vi "CRYMake CRY6181 Calibration Data.vi"() -> (0 "Error":bool)   [LabVIEW 2013]
uses:
  Typedef Control/CRYHardware Channel Info.ctl
  Typedef Control/CRYCalibration 2DCluster.ctl
  Typedef Control/CRYCalibration Cluster.ctl
  Typedef Control/CRYData Cluster.ctl
  CRYProject/CRYProject Editor Global.vi
  Calibration/SubVI/CRYCal Global.vi
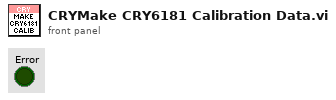
[diagram p1: front panel]
types:
  T1 = typedef "CRYCalibration 2DCluster.ctl" = cluster{"Calibration":T2, "Corr Curve":T3, "EQ Curve":T3, "Sens Curve":T3}
  T2 = typedef "CRYCalibration Cluster.ctl" = cluster{"Calibration Step Name":string, "Device":string, "Correction Curve Name":string, "Equalization Curve Name":string, "Sensitivity Curve Name":string, "Corr Folder and File":string, "EQ Folder and File":string, "Sens Folder and File":string, "Corr Step size":u16, "EQ Step size":u16, "Input":bool, "Last Cal Date (sec)":timestamp, "Cha Name":string, "Corr Curve Found":bool, "EQ Curve Found":bool, "Sens Curve Found":bool, "Signal Type":string, "Calibrated Device":string, "Hz":u32}
  T3 = typedef "CRYData Cluster.ctl" = cluster{"Name":string, "Curve":cluster{"x":dbl, "y":dbl, "z":dbl}[], "X data":u16, "Y data":u16, "Z data":u16, "X axis":u16, "Y axis":u16, "Z axis":u16, "X unit":string, "Y unit":string, "Z unit":string, "X dB ref":dbl, "Y dB ref":dbl, "Z dB ref":dbl, "single val":bool, "protected":bool, "display X":bool, "display Y":bool, "display Z":bool, "Test Info":string, "Step No.":i32, "Plot Settings":cluster{"Color":u32, "Interpolation":u8, "Point Style":u8, "Line Style":u8, "Point Color":u32, "Line Width":u8, "Bar Plot Style":u8, "Fill To":i16}, "AutoProtect":bool}
  T4 = typedef "CRYHardware Channel Info.ctl" = cluster{"ID":i32, "Name":string, "Digital":bool, "Input":bool, "Device Name":string, "Hardware Ch ID":u8, "Vmax (V)":dbl, "Latency (samples)":dbl, "Sampling Rate (Hz)":u32, "Bit Depth":u32, "Anti-aliasing Factor (%fs)":sgl, "DAQmx Channel":tag, "term config":i32, "Coupling":i32, "IEPE en":bool, "ASIOChannel Name":string, "Audio Driver":u16, "ASIOChannel Index":u8}
  T5 = typedef "CRYStep.ctl" = cluster{"No.VI":i32, "Category":string, "StepName":string, "Seq setup flattened":string, "Comment":string, "Steps config.":bool[], "Jump config":i32[], "Start":dbl, "Increment":dbl, "Name":string, "Unit":string, "Y data":u16, "Y prefix":string, "Y dB ref":dbl, "Y unit":string, "Repeat State Array":cluster{"Start":dbl, "Increment":dbl, "Count":i32, "Num":i32}[]}
  T6 = typedef "CRYCalibration All Cluster.ctl" = cluster{"Calibration 2D":T1[], "Help":string, "Tab Value":i32, "Input Signal Type":string, "Output Signal Type":string}
  T7 = typedef "CRYHardware.ctl" = cluster{"Name":string, "Analog I/O":u16, "Digital I/O":u16, "Channels":u8, "Dig Dev ID":u8, "N ports":u8, "Interface":u32, "Dig I/O Ports":cluster{"port #":i16, "width":i16, "direction":i32}[], "Interf settings":cluster{"Type":u16, "COM Port":u8, "Baud rate":u32, "Data bits":u32, "Parity":u16, "Stop bits":u16, "Flow control":u16, "Dev ID IEEE":u8}[], "N interfs":i32, "udev SNs":i16[], "udev enable":bool, "Channel Array":T4[], "Cal sequence":string, "SelectedIn":u16, "SelectedOut":u16, "SelectedTab":u16, "State":bool, "Help":string, "Advanced":bool, "In Audio Driver":u16, "Out Audio Driver":u16}
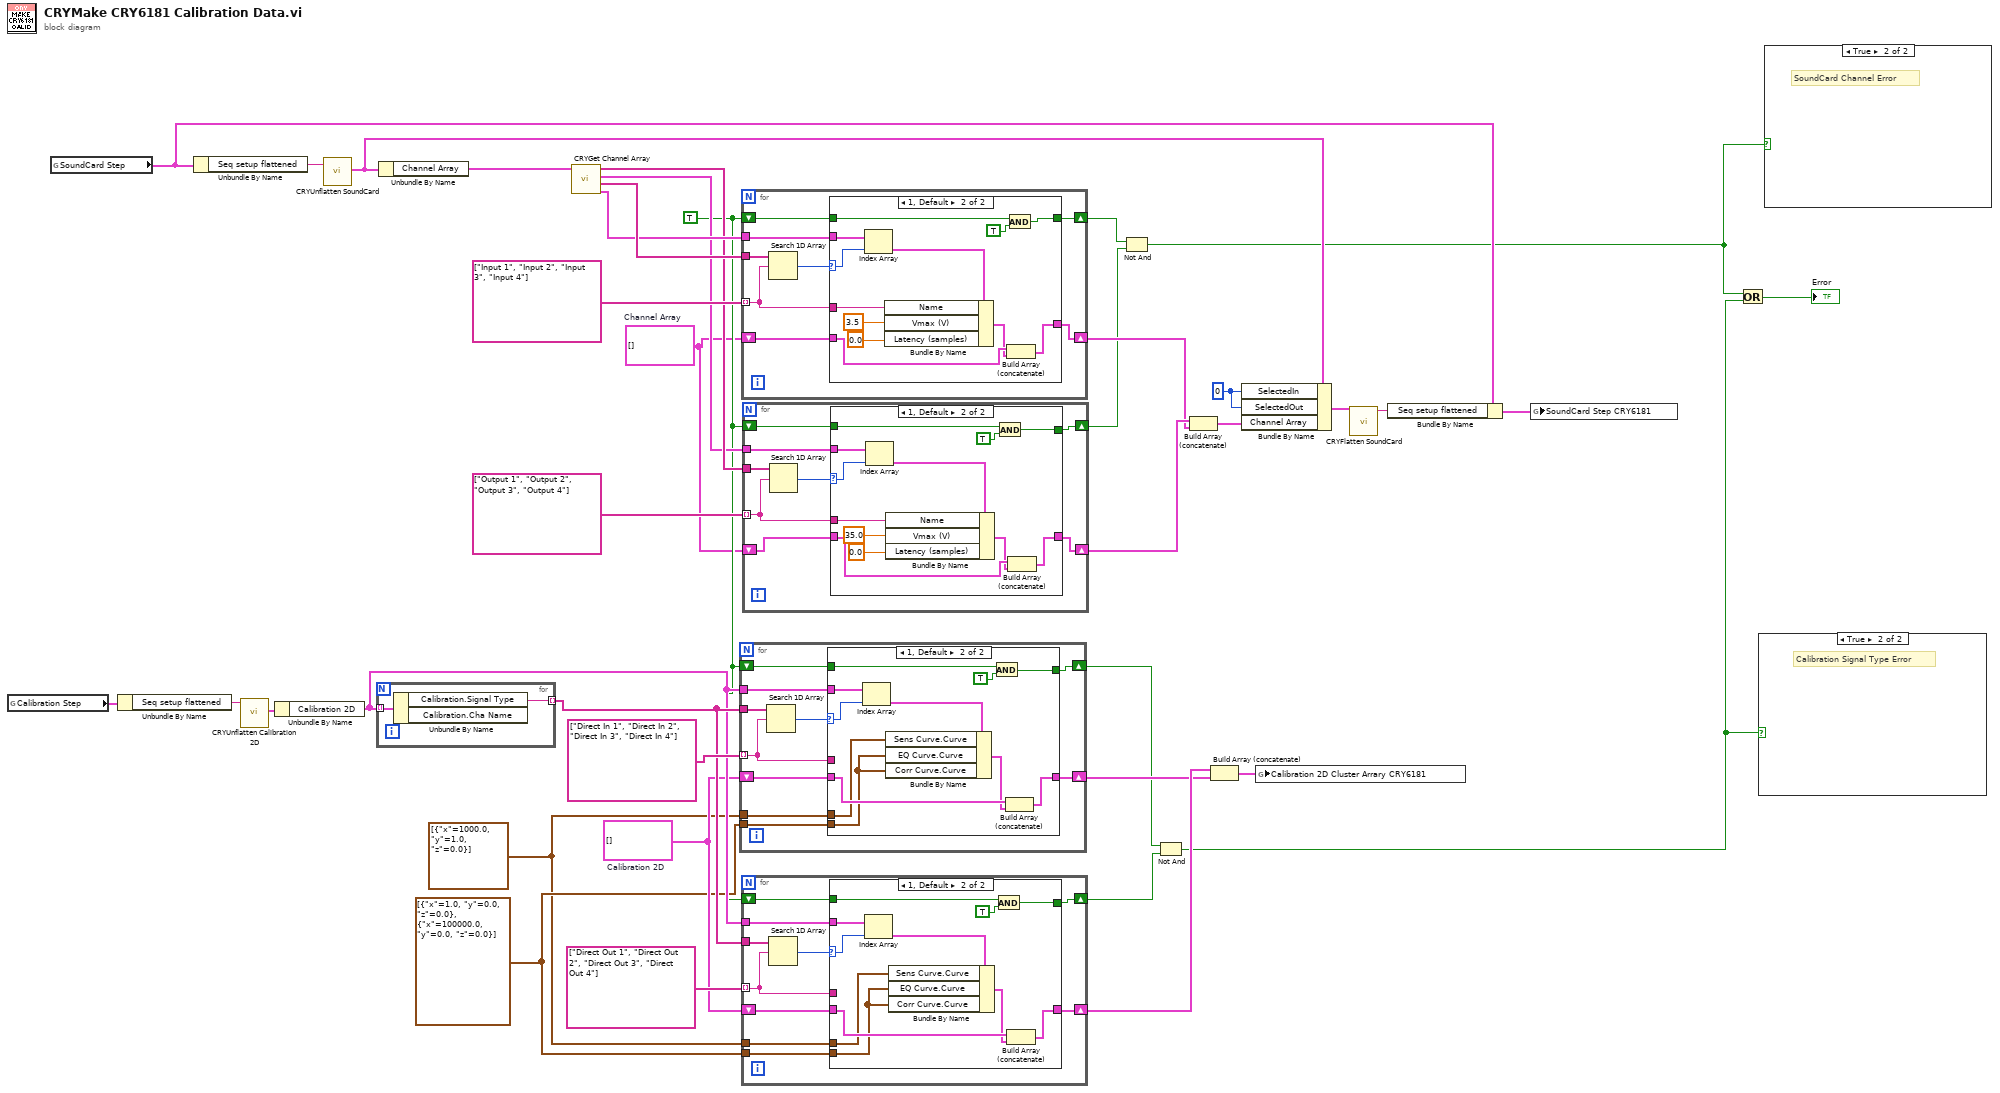
[diagram p0: block diagram]
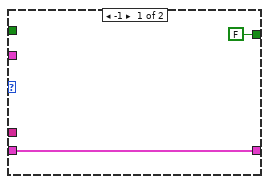
[diagram p4: hidden frame]
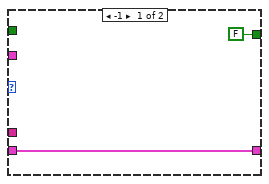
[diagram p5: hidden frame]
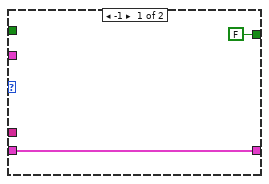
[diagram p6: hidden frame]
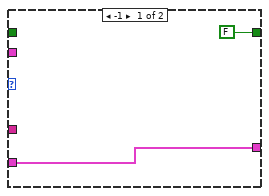
[diagram p7: hidden frame]
diagram:
  w10 = cluster{"x":dbl, "y":dbl, "z":dbl}[] [{"x"=1.0, "y"=0.0, "z"=0.0}, {"x"=100000.0, "y"=0.0, "z"=0.0}] ("EQ Curve.Curve")
  w9 = cluster{"x":dbl, "y":dbl, "z":dbl}[] [{"x"=1000.0, "y"=1.0, "z"=0.0}] ("Sens Curve.Curve")
  w13 = T1[] []  # Calibration 2D
  w2 = TRUE
  w29 = u16 0 ("SelectedIn")
  w1 = T4[] []  # Channel Array
  n1 = global read "CRYProject Editor Global.vi" "Calibration Step"() -> (w17:T5)
  n2 = global read "CRYProject Editor Global.vi" "SoundCard Step"() -> (w23:T5)
  n3 = Unbundle By Name(w17) -> ("Seq setup flattened"=w20:string)
  n4 = Unbundle By Name(w23) -> ("Seq setup flattened"=w24:string)
  n5 = call "CRYUnflatten Calibration 2D.vi"("Flattened Calibration"=w20) -> ("Calibration Step Out"=w18:T6)  [unwired: 8 in, 2 out]
  n6 = Unbundle By Name(w18) -> ("Calibration 2D"=w14:T1[])
  n7 = call "CRYUnflatten SoundCard.vi"("Flatten SoundCard"=w24) -> ("SoundCard"=w25:T7)  [unwired: 8 in, 2 out]
  n8 = for {
    tunnel: w14 -> [w41] mode=indexing
    tunnel: [w40] -> w15 mode=indexing
    n9 = Unbundle By Name(w41) -> ("Calibration.Signal Type"=w40:string)  [unwired: 1 out]
  }
  n10 = Unbundle By Name(w25) -> ("Channel Array"=w38:T4[])
  n11 = call "CRYGet Channel Array.vi"("Channel Array"=w38) -> ("I Channel Info Out"=w36:T4[], "I_Channel Name Out"=w37:string[], "O Channel Info Out"=w33:T4[], "O_Channel Name Out"=w34:string[])  [unwired: 7 in]
  n12 = for {
    tunnel: string[] ["Direct In 1", "Direct In 2", "Direct In 3", "Direct In 4"] -> [w49] mode=indexing
    tunnel: w15 -> [w50]
    tunnel: w14 -> [w47]
    shift-right: [w51] -> w11
    shift-left: w13 -> [w46]
    shift-right: [w44] -> w8
    shift-left: w2 -> [w45]
    tunnel: w9 -> [w43]
    tunnel: w10 -> [w42]
    n13 = Search 1D Array(1D array=w50, element=w49) -> (index of element=w48:i32)  [unwired: 1 in]
    n14 = case shown="1, Default" w48 {
      selector: w48 -> [_ w63]
      tunnel: [w53 w61] -> w51
      tunnel: w49 -> [_ _]
      tunnel: w47 -> [_ w64]
      tunnel: w46 -> [w53 w62]
      tunnel: w45 -> [_ w59]
      tunnel: [FALSE w58] -> w44
      tunnel: w43 -> [_ w55]
      tunnel: w42 -> [_ w54]
      frame -1 {
      }
      frame 1, Default {
        n15 = Index Array(array=w64, index=w63) -> (element=w57:T1)
        n16 = Bundle By Name(cluster=w57, "Sens Curve.Curve"=w55, "EQ Curve.Curve"=w54, "Corr Curve.Curve"=w54) -> (w56:T1)
        n17 = And(x=w59, y=TRUE) -> (x .and. y?=w58:bool)
        n18 = Build Array (concatenate)(w62, w56) -> (w61:T1[])
      }
    }
  }
  n19 = for {
    tunnel: string[] ["Input 1", "Input 2", "Input 3", "Input 4"] -> [w70] mode=indexing
    tunnel: w37 -> [w71]
    tunnel: w36 -> [w68]
    shift-right: [w72] -> w31
    shift-left: w1 -> [w67]
    shift-right: [w65] -> w21
    shift-left: w2 -> [w66]
    n20 = Search 1D Array(1D array=w71, element=w70) -> (index of element=w69:i32)  [unwired: 1 in]
    n21 = case shown="1, Default" w69 {
      selector: w69 -> [_ w82]
      tunnel: [w74 w78] -> w72
      tunnel: w70 -> [_ w84]
      tunnel: w68 -> [_ w83]
      tunnel: w67 -> [w74 w80]
      tunnel: w66 -> [_ w77]
      tunnel: [FALSE ("x .and. y?") w75] -> w65
      frame -1 {
      }
      frame 1, Default {
        n22 = Index Array(array=w83, index=w82) -> (element=w81:T4)
        n23 = Bundle By Name(cluster=w81, "Name"=w84, "Vmax (V)"=3.5, "Latency (samples)"=0.0 ("Vmax (V)")) -> (w79:T4)
        n24 = And(x=w77, y=TRUE) -> (x .and. y?=w75:bool)
        n25 = Build Array (concatenate)(w80, w79) -> (w78:T4[])
      }
    }
  }
  n26 = for {
    tunnel: string[] ["Direct Out 1", "Direct Out 2", "Direct Out 3", "Direct Out 4"] -> [w94] mode=indexing
    tunnel: w15 -> [w95]
    tunnel: w14 -> [w92]
    shift-right: [w96] -> w12
    shift-left: w13 -> [w91]
    shift-right: [w89] -> w7
    shift-left: w2 -> [w90]
    tunnel: w10 -> [w88]
    tunnel: w9 -> [w87]
    n27 = Search 1D Array(1D array=w95, element=w94) -> (index of element=w93:i32)  [unwired: 1 in]
    n28 = case shown="1, Default" w93 {
      selector: w93 -> [_ w108]
      tunnel: [w98 w106] -> w96
      tunnel: w94 -> [_ _]
      tunnel: w92 -> [_ w109]
      tunnel: w91 -> [w98 w107]
      tunnel: w90 -> [_ w104]
      tunnel: [FALSE w103] -> w89
      tunnel: w88 -> [_ w100]
      tunnel: w87 -> [_ w99]
      frame -1 {
      }
      frame 1, Default {
        n29 = Index Array(array=w109, index=w108) -> (element=w102:T1)
        n30 = Bundle By Name(cluster=w102, "Sens Curve.Curve"=w99, "EQ Curve.Curve"=w100, "Corr Curve.Curve"=w100) -> (w101:T1)
        n31 = And(x=w104, y=TRUE) -> (x .and. y?=w103:bool)
        n32 = Build Array (concatenate)(w107, w101) -> (w106:T1[])
      }
    }
  }
  n33 = for {
    tunnel: string[] ["Output 1", "Output 2", "Output 3", "Output 4"] -> [w115] mode=indexing
    tunnel: w34 -> [w116]
    tunnel: w33 -> [w113]
    shift-right: [w117] -> w32
    shift-left: w1 -> [w112]
    shift-right: [w110] -> w22
    shift-left: w2 -> [w111]
    n34 = Search 1D Array(1D array=w116, element=w115) -> (index of element=w114:i32)  [unwired: 1 in]
    n35 = case shown="1, Default" w114 {
      selector: w114 -> [_ w127]
      tunnel: [w119 w123] -> w117
      tunnel: w115 -> [_ w129]
      tunnel: w113 -> [_ w128]
      tunnel: w112 -> [w119 w125]
      tunnel: w111 -> [_ w121]
      tunnel: [FALSE w120] -> w110
      frame -1 {
      }
      frame 1, Default {
        n36 = Index Array(array=w128, index=w127) -> (element=w126:T4)
        n37 = Bundle By Name(cluster=w126, "Name"=w129, "Vmax (V)"=35.0, "Latency (samples)"=0.0 ("Vmax (V)")) -> (w124:T4)
        n38 = And(x=w121, y=TRUE) -> (x .and. y?=w120:bool)
        n39 = Build Array (concatenate)(w125, w124) -> (w123:T4[])
      }
    }
  }
  n40 = Not And(1:w22, 2:w21) -> (0:w4:bool)
  n41 = Not And(1:w7, 2:w8) -> (0:w5:bool)
  n42 = Build Array (concatenate)(w32, w31) -> (w30:T4[])
  n43 = Build Array (concatenate)(w12, w11) -> (w6:T1[])
  n44 = Bundle By Name(cluster=w25, "SelectedIn"=w29, "SelectedOut"=w29, "Channel Array"=w30) -> (w28:T7)
  n45 = global write "CRYCal Global.vi" "Calibration 2D Cluster Arrary CRY6181"(w6) -> ()
  n46 = call "CRYFlatten SoundCard.vi"("SoundCard"=w28) -> ("SoundCard flattened"=w27:string)  [unwired: 10 in]
  n47 = Bundle By Name(cluster=w23, "Seq setup flattened"=w27) -> (w26:T5)
  n48 = global write "CRYCal Global.vi" "SoundCard Step CRY6181"(w26) -> ()
  n49 = Or(x=w4, y=w5) -> (x .or. y?=→"Error":bool)
  n50 = case shown="True" w5 {
    frame False {
    }
    frame True {
      # "Calibration Signal Type Error"
    }
  }
  n51 = case shown="True" w4 {
    frame False {
    }
    frame True {
      # "SoundCard Channel Error"
    }
  }
